vi "Q.Obtain Queue.vi"(4 "Init.Data2":variant, 6 "Init.Data1":variant, 7 "Enqueue Init":bool, 8 "Error In":errorcluster, 10 "Init.Sub":string, 11 "Q Name":string) -> (0 "error out":errorcluster, 2 "created new?":bool, 3 "Q Out":refnum<queue>)   [LabVIEW 2024, in "EQMF.lvlib" / "Queue Utils.lvlib"]
doc: "This VI enqueues an element to the Queue.\n\nThis VI obtains the queue by name or by queue reference.\n\nIf the 'Q Name' input is empty then it obtains the queue by the 'Q In\" reference.\nIf the 'Q Name' input is NOT empty then it obtains the queue by the this name.\n If a queue is ontained by name and the queue does not already exits, an error is generated.\n\nThe 'Top of Q' input is TRUE by default.\nThis input will cause this item to be enqueued on the top of the queue when it is TRUE."
uses:
  Queue Utils.lvlib
  Q.Element.ctl
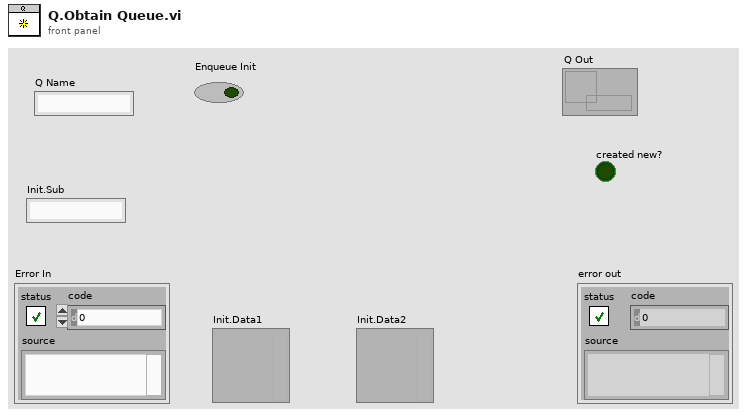
[diagram p1: front panel]
types:
  T1 = typedef "EQMF.lvlib/Queue Utils.lvlib/Q.Element.ctl" = cluster{"Cmd":string, "Sub":string, "Data1":variant, "Data2":variant}
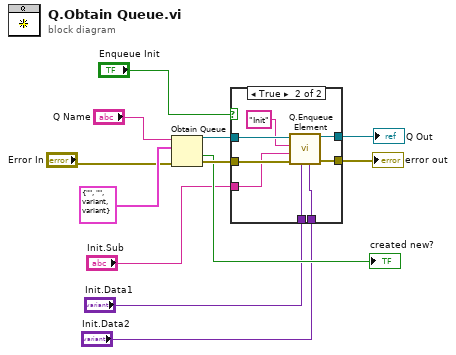
[diagram p0: block diagram]
diagram:
  n1 = Obtain Queue(name (unnamed)="Q Name", element data type=T1 {"Cmd"="", "Sub"="", "Data1"=variant, "Data2"=variant} ("Q.Element"), error in (no error)="Error In") -> (queue out=w7:refnum<queue>, created new?=→"created new?":bool, error out=w6:errorcluster)  [unwired: 2 in]
  n2 = case shown="True" "Enqueue Init" {
    tunnel: w7 -> [w14 w22]
    tunnel: w6 -> [w13 w21]
    tunnel: [w14 w20] -> w12
    tunnel: [w13 w19] -> w11
    tunnel: "Init.Sub" -> [_ w17]
    tunnel: "Init.Data1" -> [_ w16]
    tunnel: "Init.Data2" -> [_ w15]
    frame False {
    }
    frame True {
      n3 = call "Q.Enqueue Element.vi"("Data2"=w15, "Data1"=w16, "error in"=w21, "Sub"=w17, "Cmd"="Init", "Q In"=w22) -> ("error out"=w19:errorcluster, "Q Out"=w20:refnum<queue>)  [unwired: 4 in]
    }
  }
  "error out" <- w11
  "Q Out" <- w12
